vi "EventStructure.vi"() -> ()   [LabVIEW 2020]
uses:
  <vilib>/event_ctls.llb/lveventtype.ctl
  <vilib>/event_ctls.llb/eventsource.ctl
panel:
  out "LoopCount":i32
  out "CtlRef":string
  out "Button OldVal":bool
  out "ButtonTime":u32
  out "ButtonSource":T1 items=["LabVIEW UI"=0, "ActiveX"=1, "User Event"=25]
  out "ButtonType":T2=enum."Value Change"
  out "Button NewVal":bool
  in  "Button":bool
  out "TImeoutTime":u32
  out "TimeoutSource":T1 items=["LabVIEW UI"=0, "ActiveX"=1, "User Event"=25]
  in  "stop":bool
  out "TimeoutType":T2=enum."Value Change"
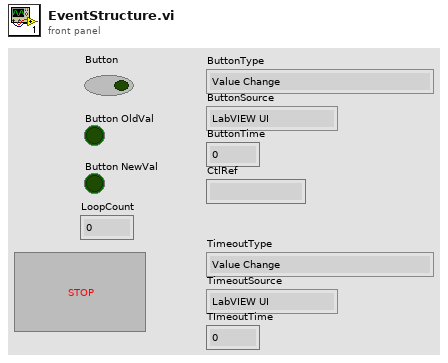
[diagram p1: front panel]
types:
  T1 = typedef "eventsource.ctl" = u32
  T2 = typedef "lveventtype.ctl" = enum32{"Null", "Timeout", "Annotation Menu Selection", "Annotation Menu Selection?", "App Instance Close", "App Instance Close?", "Autoscale Range Change", "Bookmark Info Change", "Cell Edit", "Cell Edit?", "Cursor Grab", "Cursor Grab?", "Cursor Menu Selection", "Cursor Menu Selection?", "Cursor Move", "Cursor Release", "Data Change", "Direction Change", "Display State Change", "Drag Ended", "Drag Enter", "Drag Leave", "Drag Over", "Drag Source Update", "Drag Starting", "Drag Starting?", "Drop", "Exec State Change", "Key Down", "Key Down?", "Key Repeat", "Key Repeat?", "Key Up", "Listbox Double Click", "Menu Activation?", "Menu Selection (App)", "Menu Selection? (App)", "Menu Selection (User)", "Mouse Down", "Mouse Down?", "Mouse Enter", "Mouse Leave", "Mouse Move", "Mouse Up", "Mouse Wheel", "NI Security User Change (App)", "Pane Size", "Panel Close", "Panel Close?", "Panel Resize", "Plot Attribute Change", "Scale Range Change", "Shortcut Menu Activation?", "Shortcut Menu Selection (App)", "Shortcut Menu Selection? (App)", "Shortcut Menu Selection (User)", "Tree Double Click", "Tree Drag", "Tree Drag?", "Tree Drop", "Tree Drop?", "Tree Item Close", "Tree Item Close?", "Tree Item Open", "Tree Item Open?", "User Event", "Value Change"}
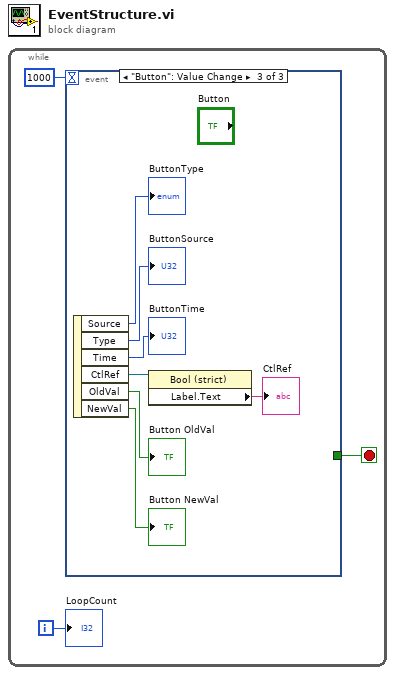
[diagram p0: block diagram]
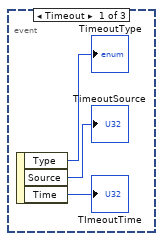
[diagram p2: hidden frame]
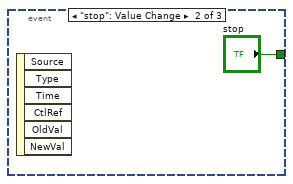
[diagram p3: hidden frame]
diagram:
  n1 = while {
    i -> [w1]
    stop <- w3 stop-if-true
    n2 = event shown="[2] \"Button\": Value Change" {
      selector: _ -> [_ _ _]
      dyn-events: _ -> [_ _ _]
      timeout: 1000 -> [_ _ _]
      tunnel: [_ "stop" _] -> w3
      event Timeout {
        n3 = event-data() -> ("Type"=→"TimeoutType":T2, "Source"=→"TimeoutSource":T1, "Time"=→"TImeoutTime":u32)  [unwired: 1 in]
      }
      event "stop": Value Change {
        n4 = event-data() -> ()  [unwired: 1 in, 6 out]
      }
      event "Button": Value Change {
        n5 = event-data() -> ("Source"=→"ButtonType":T1, "Type"=→"ButtonSource":T2, "Time"=→"ButtonTime":u32, "CtlRef"=w9:refnum<vi>, "OldVal"=→"Button OldVal":bool, "NewVal"=→"Button NewVal":bool)  [unwired: 1 in]
        n6 = property class="Bool (strict)"(reference=w9) -> ("Label.Text"=→"CtlRef":string)  [unwired: 1 in, 2 out]
      }
    }
    "LoopCount" <- w1
  }
